vi "Configure GPIO Pin.vi"(0 "VISA resource name":refnum<visa-resource-name>, 2 "GPIO Pin Trigger Timing (2: Both)":i32(ring)=2 items=["Before", "After", "Both"], 3 "GPIO Pin Trigger PW (0.0001 seconds)":dbl=0.0001, 5 "Pin Number (1)":i32=1, 7 "GPIO Pin Polarity (0: Positive)":i32(ring) items=["Positive", "Negative"], 9 "GPIO Pin I/O Function (0: DINP)":i32(ring) items=["DINP", "DIO", "HVOL", "TINP", "TOUT"], 11 "error in (no error)":errorcluster, 13 "GPIO Pin Trigger Type (0: Edge)":i32(ring) items=["Edge", "Level"]) -> (4 "VISA resource name out":refnum<visa-resource-name>, 15 "error out":errorcluster)   [LabVIEW 2020, in "Agilent B2900 Series.lvlib"]
doc: "Configure GPIO(General Purpose I/O) Pin, which is an I/O port of the Digital I/O D-sub connector on the rear panel. Can be used as\ntrigger input/output terminals or as an interface to a handler or the likes."
uses:
  Agilent B2900 Series.lvlib
panel:
  # "GPIO Pin Trigger Settings"
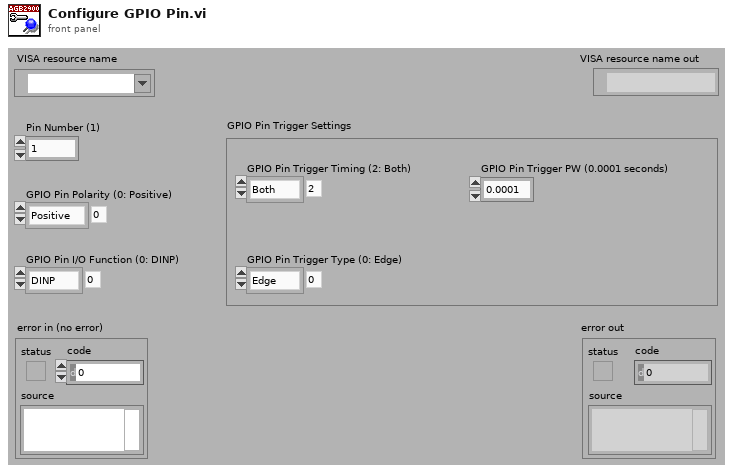
[diagram p1: front panel]
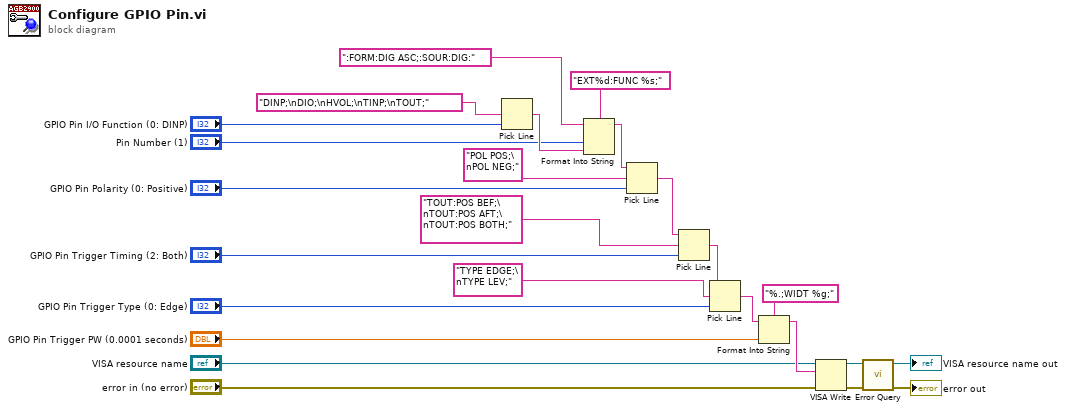
[diagram p0: block diagram]
diagram:
  n1 = Pick Line(multi-line string="DINP;\nDIO;\nHVOL;\nTINP;\nTOUT;", line index="GPIO Pin I/O Function (0: DINP)") -> (output string=w4:string)  [unwired: 1 in]
  n2 = Format Into String(format string="EXT%d:FUNC %s;", initial string=":FORM:DIG ASC;:SOUR:DIG:", "Pin Number (1)", w4) -> (resulting string=w2:string)  [unwired: 1 in, 1 out]
  n3 = Pick Line(string ("")=w2, multi-line string="POL POS;\nPOL NEG;", line index="GPIO Pin Polarity (0: Positive)") -> (output string=w19:string)
  n4 = Pick Line(string ("")=w19, multi-line string="TOUT:POS BEF;\nTOUT:POS AFT;\nTOUT:POS BOTH;", line index="GPIO Pin Trigger Timing (2: Both)") -> (output string=w16:string)
  n5 = Pick Line(string ("")=w16, multi-line string="TYPE EDGE;\nTYPE LEV;", line index="GPIO Pin Trigger Type (0: Edge)") -> (output string=w15:string)
  n6 = Format Into String(format string="%.;WIDT %g;", initial string=w15, "GPIO Pin Trigger PW (0.0001 seconds)") -> (resulting string=w12:string)  [unwired: 1 in, 1 out]
  n7 = VISA Write(VISA resource name="VISA resource name", write buffer=w12, error in (no error)="error in (no error)") -> (VISA resource name out=w9:refnum<visa-resource-name>, error out=w8:errorcluster)  [unwired: 1 out]
  n8 = call "Error Query.vi"("error in (no error)"=w8, "VISA resource name"=w9) -> ("error out"=→"error out":errorcluster, "VISA resource name out"=→"VISA resource name out":refnum<visa-resource-name>)  [unwired: 6 in, 2 out]
